vi "niFpgaInitialConditionTemplate.vi"(0 "input":fxp<+/-,16,16>, 1 "reset":bool, 7 "initial condition":fxp<+/-,32,32>) -> (4 "output":fxp<+/-,32,32>)   [LabVIEW 2017]
doc: "Produces a predefined initial condition immediately after the first time you call or initialize the VI. The data type you wire to <B>input</B> determines the <B>output</B> data type."
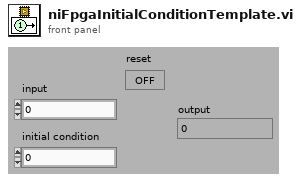
[diagram p1: front panel]
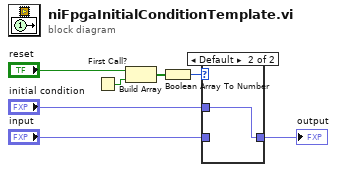
[diagram p0: block diagram]
diagram:
  n1 = First Call?() -> (First Call?: T/F=w3:bool)
  n2 = Build Array("reset", w3) -> (w2:bool[])
  n3 = Boolean Array To Number(Boolean array=w2) -> (number=w7:u8)
  n4 = case shown="Default" w7 {
    tunnel: "input" -> [w8 _]
    tunnel: [w8 w9] -> w5
    tunnel: "initial condition" -> [_ w9]
    frame 0 {
    }
    frame Default {
    }
  }
  "output" <- w5
